vi "CPP-FFIDsimpleBG.vi"() -> (0 "New Values In":string[][](array[string]), 1 "New Chs In":string[](array[string]))   [LabVIEW 2020]
uses:
  d07341dc-eb23-f54f-b463-cf807e562f07.vi
  Results_plotter_Global.vi
  Data plotting/subVIs/Plot_Values_Global.vi
panel:
  in  "MaxBGinterval(min)":dbl=35.0
  in  "MaxBGdelta(ppm)":dbl=40.0
  in  "Mode":bool
  out "C-BG":dbl[](array[numeric])
  out "BGs":dbl[](array[numeric]) format="%#.1g"
  out "AllValues":dbl[](array[numeric])
  out "AllTimes":dbl[](array[numeric])
  out "BGvalues":dbl[](array[numeric]) format="%#.2f"
  out "BGtimes":dbl[](array[numeric])
  out "legends":string[](array[string])
  out "plottedChannel":string[](array[string])
  # "Instructions:\nPlot the  original Mean Concentration for the files you want correcting and the FF_Bkgnd_Info file(s) stored alongside them. Call this VI with the \"Calculate new metadata\" button on the Edit tab. This VI will interpolate the background values, and subtract them from the original concentrations"
  # "https://wiki.4winds.tools/index.php/14256-_BOEM-_Offshore_Structure_Wakes_with_Omniprobe_and_FastFID?venotify=created#Instructions_for_use"
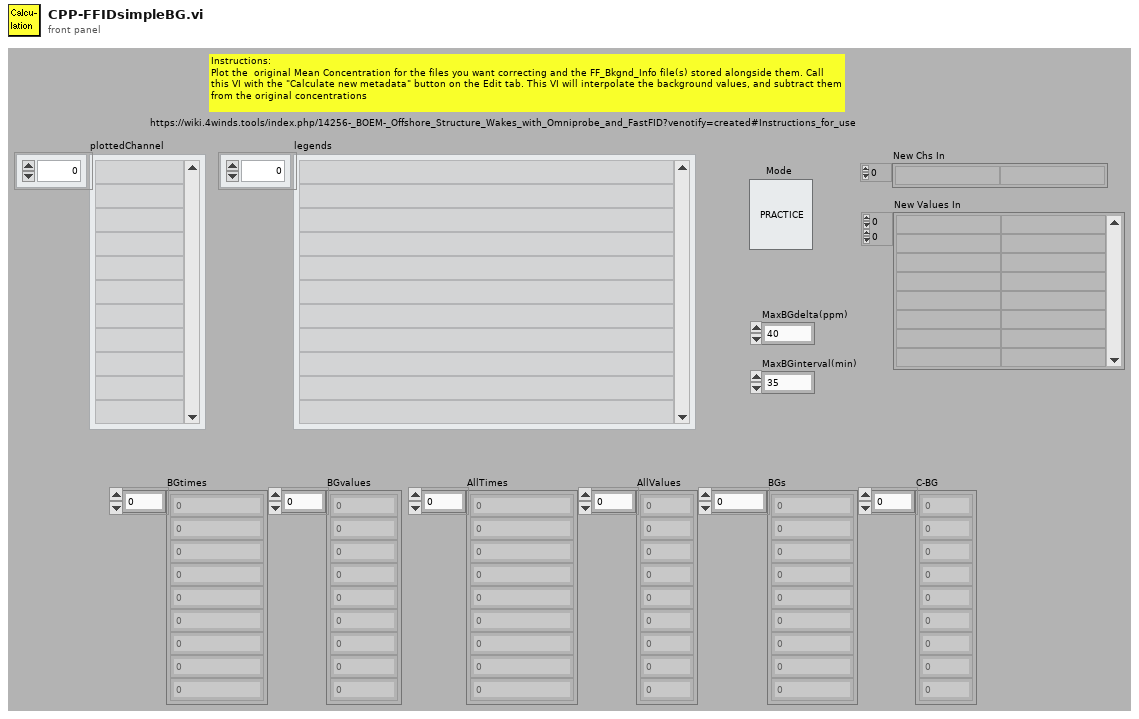
[diagram p1: front panel]
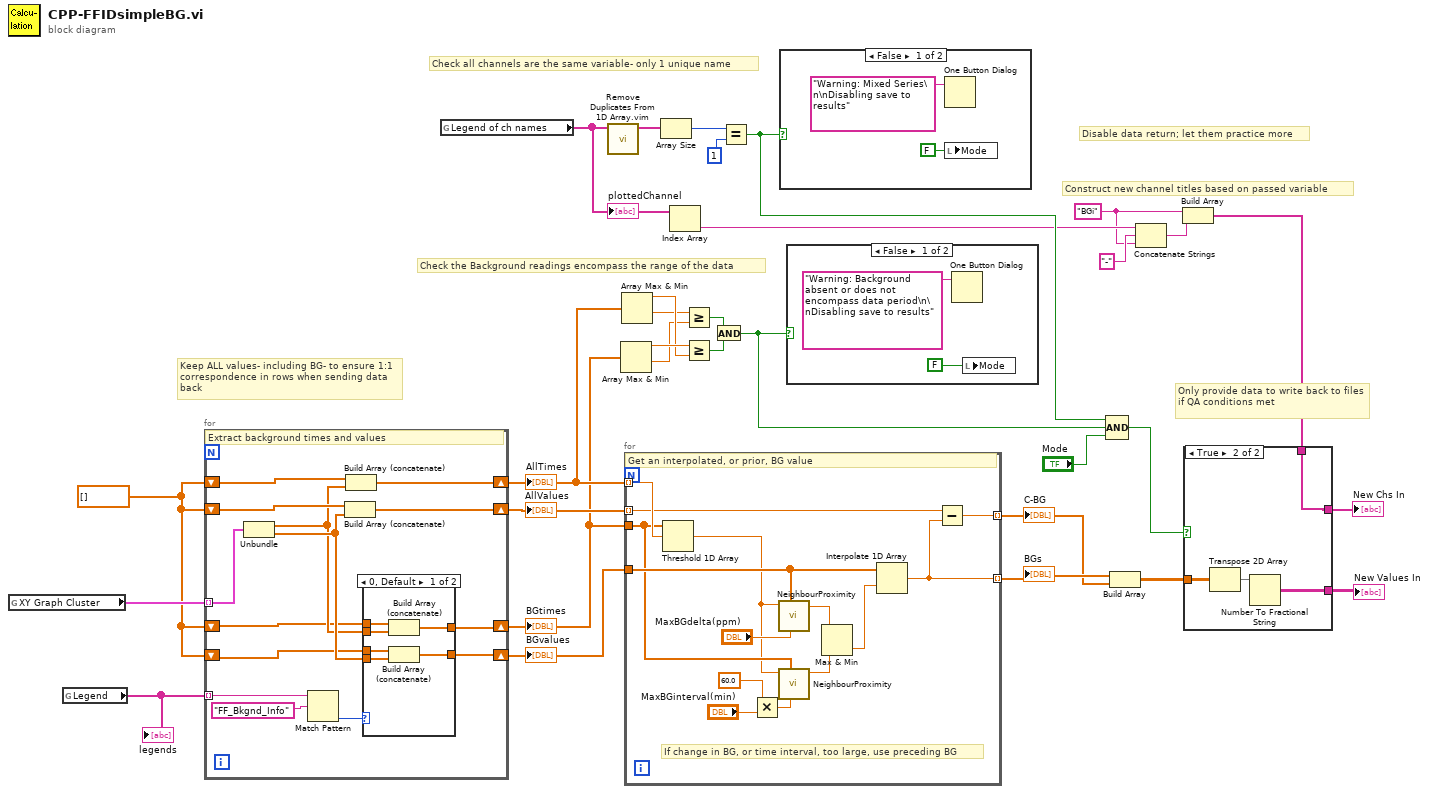
[diagram p0: block diagram]
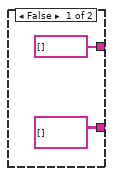
[diagram p4: hidden frame]
diagram:
  w5 = "BGi"
  w1 = dbl[] []
  # "Construct new channel titles based on passed variable"
  # "Disable data return; let them practice more"
  # "Keep ALL values- including BG- to ensure 1:1 correspondence in rows when sending data back"
  # "Only provide data to write back to files if QA conditions met"
  # "Check the Background readings encompass the range of the data"
  # "Check all channels are the same variable- only 1 unique name"
  n1 = global read "Plot_Values_Global.vi" "XY Graph Cluster"() -> (w30:cluster{dbl[], dbl[]}[])
  n2 = global read "Results_plotter_Global.vi" "Legend"() -> (w31:string[])
  "legends" <- w31
  n3 = for {
    tunnel: w31 -> [w45] mode=indexing
    tunnel: w30 -> [w42] mode=indexing
    shift-right: [w40] -> w18
    shift-left: w1 -> [w39]
    shift-right: [w34] -> w29
    shift-left: w1 -> [w32]
    shift-right: [w41] -> w28
    shift-left: w1 -> [w38]
    shift-right: [w35] -> w17
    shift-left: w1 -> [w33]
    # "Extract background times and values"
    n4 = Unbundle(w42) -> (w36:dbl[], w37:dbl[])
    n5 = Match Pattern(string=w45, regular expression="FF_Bkgnd_Info") -> (offset past match=w43:i32)  [unwired: 1 in, 3 out]
    n6 = Build Array (concatenate)(w38, w37) -> (w41:dbl[])
    n7 = Build Array (concatenate)(w39, w36) -> (w40:dbl[])
    n8 = case shown="0, Default" w43 {
      tunnel: w37 -> [w51 _]
      tunnel: w36 -> [w50 _]
      tunnel: [w49 w53] -> w35
      tunnel: [w48 w52] -> w34
      tunnel: w33 -> [w47 w53]
      tunnel: w32 -> [w46 w52]
      frame 0, Default {
        n9 = Build Array (concatenate)(w47, w50) -> (w49:dbl[])
        n10 = Build Array (concatenate)(w46, w51) -> (w48:dbl[])
      }
      frame -1 {
      }
    }
  }
  "BGtimes" <- w17
  "BGvalues" <- w29
  "AllTimes" <- w18
  "AllValues" <- w28
  n11 = global read "Results_plotter_Global.vi" "Legend of ch names"() -> (w8:string[])
  "plottedChannel" <- w8
  n12 = call "Remove Duplicates From 1D Array.vim"("array"=w8) -> ("array with duplicates removed"=w22:string[])  [unwired: 10 in]
  n13 = Array Max & Min(array=w17) -> (max value=w16:dbl, min value=w14:dbl)  [unwired: 2 out]
  n14 = Array Max & Min(array=w18) -> (max value=w15:dbl, min value=w13:dbl)  [unwired: 2 out]
  n15 = for {
    tunnel: w18 -> [w67] mode=indexing
    tunnel: w17 -> [w61]
    tunnel: w29 -> [w63]
    tunnel: [w64] -> w27 mode=indexing
    tunnel: [w65] -> w26 mode=indexing
    tunnel: w28 -> [w66] mode=indexing
    # "If change in BG, or time interval, too large, use preceding BG"
    # "Get an interpolated, or prior, BG value"
    n16 = Threshold 1D Array(2:w67, 3:w61) -> (0:w60:dbl)  [unwired: 1 in]
    n17 = Multiply(x=60.0, y="MaxBGinterval(min)") -> (x*y=w58:dbl)
    n18 = call "NeighbourProximity.vi"("MaxInterval"="MaxBGdelta(ppm)", "Values"=w63, "InterpolatedIndex"=w60) -> ("IndexToUse"=w56:dbl)  [unwired: 7 in, 1 out]
    n19 = call "NeighbourProximity.vi"("MaxInterval"=w58, "Values"=w61, "InterpolatedIndex"=w60) -> ("IndexToUse"=w55:dbl)  [unwired: 7 in, 1 out]
    n20 = Max & Min(x=w56, y=w55) -> (min(x,y)=w54:dbl)  [unwired: 1 out]
    n21 = Interpolate 1D Array(1:w54, 2:w63) -> (0:w64:dbl)
    n22 = Subtract(x=w66, y=w64) -> (x-y=w65:dbl)
  }
  "BGs" <- w27
  "C-BG" <- w26
  n23 = Array Size(array=w22) -> (size(s)=w21:i32)
  n24 = Index Array(array=w8) -> (element=w7:string)  [unwired: 1 in]
  n25 = Greater Or Equal?(x=w13, y=w14) -> (x >= y?=w12:bool)
  n26 = Greater Or Equal?(x=w16, y=w15) -> (x >= y?=w11:bool)
  n27 = And(x=w12, y=w11) -> (x .and. y?=w9:bool)
  n28 = Equal?(x=w21, y=1) -> (x = y?=w10:bool)
  n29 = case shown="False" w10 {
    frame False {
      n30 = One Button Dialog(message="Warning: Mixed Series\n\nDisabling save to results") -> ()  [unwired: 1 in, 1 out]
      n31 = local write "Mode"(FALSE ("Mode")) -> ()
    }
    frame True {
    }
  }
  n32 = case shown="False" w9 {
    frame False {
      n33 = One Button Dialog(message="Warning: Background absent or does not encompass data period\n\nDisabling save to results") -> ()  [unwired: 1 in, 1 out]
      n34 = local write "Mode"(FALSE ("Mode")) -> ()
    }
    frame True {
    }
  }
  n35 = Compound Arithmetic op=AND(w10, w9, "Mode") -> (w19:bool)
  n36 = Build Array(w27, w26) -> (w25:dbl[][])
  n37 = Concatenate Strings(w7, "-" ("string"), w5) -> (w4:string)
  n38 = Build Array(w5, w4) -> (w3:string[])
  n39 = case shown="True" w19 {
    tunnel: w25 -> [_ w77]
    tunnel: [string[][] [] w76] -> w24
    tunnel: [string[] [] ("New Chs In") w74] -> w2
    tunnel: w3 -> [_ w74]
    frame False {
    }
    frame True {
      n40 = Transpose 2D Array(2D array=w77) -> (transposed array=w75:dbl[][])
      n41 = Number To Fractional String(number=w75) -> (F-format string=w76:string[][])  [unwired: 3 in]
    }
  }
  "New Chs In" <- w2
  "New Values In" <- w24
